vi "Read Image Blocks (SubVI).vi"(8 "Num of Image Blocks":i32, 10 "Image In":u8[][](array[numeric]), 11 "File REF In":refnum<file>) -> (2 "Image Out":u8[][](array[numeric]), 3 "File REF Out":refnum<file>)   [LabVIEW 2015]
panel:
  out "Image":T1(plugin-control)
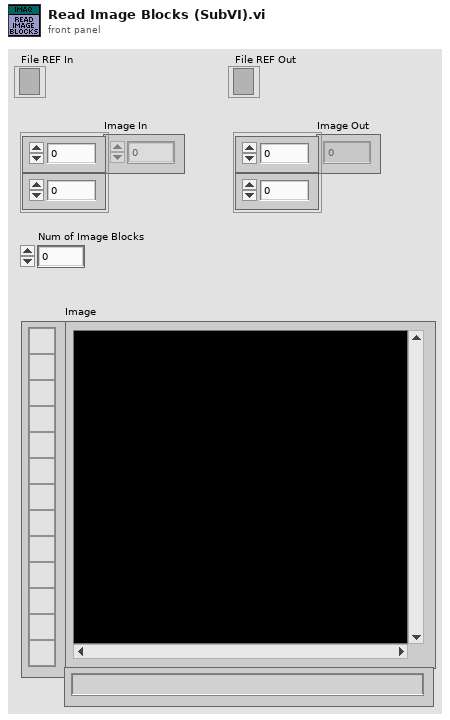
[diagram p1: front panel]
types:
  T1 = typedef "IMAQ Image.ctl" = refnum<image>
  T2 = enum16{"big-endian, network order", "native, host order", "little-endian"}
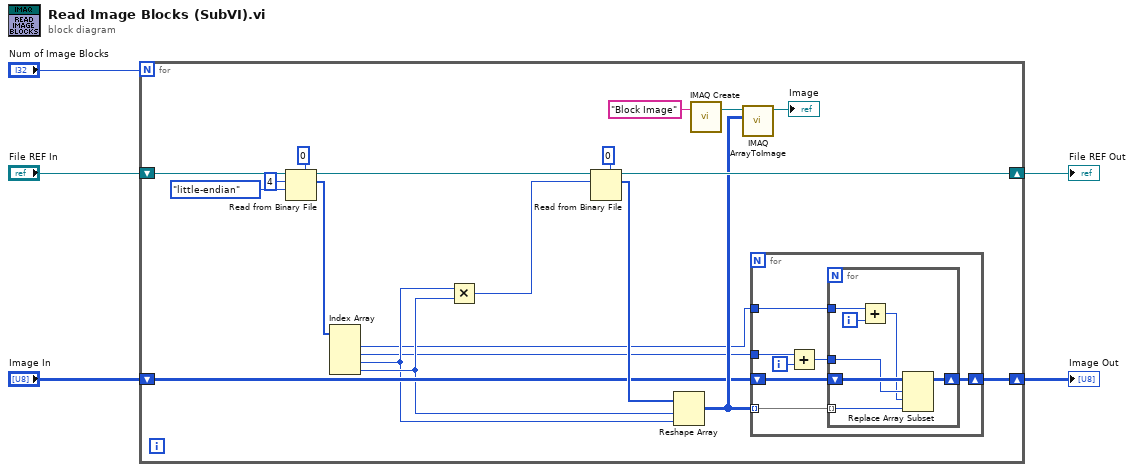
[diagram p0: block diagram]
diagram:
  n1 = for {
    N: "Num of Image Blocks" -> [_]
    shift-right: [w15] -> w2
    shift-left: "File REF In" -> [w17]
    shift-right: [w16] -> w4
    shift-left: "Image In" -> [w10]
    n2 = Read from Binary File(5:0, 9:T2."little-endian" ("byte order (0:big-endian, network order)"), 10:4 ("count (1)"), 11:w17) -> (2:w19:i32[], 3:w23:refnum<file>)  [unwired: 2 in, 2 out]
    n3 = Index Array(array=w19) -> (element #1=w6:i32, element #2=w7:i32, element #3=w8:i32, element #4=w9:i32)  [unwired: 4 in]
    n4 = Multiply(x=w8, y=w9) -> (x*y=w24:i32)
    n5 = Read from Binary File(5:u8 0, 10:w24, 11:w23) -> (2:w25:u8[], 3:w15:refnum<file>)  [unwired: 3 in, 2 out]
    n6 = Reshape Array(w25, w9, w8) -> (w11:u8[][])
    n7 = call "IMAQ Create"("Image Name"="Block Image") -> ("New Image"=w13:T1)  [unwired: 4 in, 1 out]
    n8 = call "IMAQ ArrayToImage"("Image Pixels (U8)"=w11, "Image"=w13) -> ("Image Out"=→"Image":T1)  [unwired: 8 in, 1 out]
    n9 = for {
      shift-right: [w31] -> w16
      shift-left: w10 -> [w32]
      tunnel: w7 -> [w30]
      tunnel: w11 -> [w27] mode=indexing
      tunnel: w6 -> [w26]
      i -> [w28]
      n10 = Add(x=w30, y=w28) -> (x+y=w29:i32)
      n11 = for {
        tunnel: w29 -> [w34]
        tunnel: w27 -> [w37] mode=indexing
        shift-right: [w38] -> w31
        shift-left: w32 -> [w39]
        tunnel: w26 -> [w35]
        i -> [w36]
        n12 = Add(x=w35, y=w36) -> (x+y=w33:i32)
        n13 = Replace Array Subset(array=w39, new element=w37, index (row)=w34, index (col)=w33) -> (w38:u8[][])
      }
    }
  }
  "Image Out" <- w4
  "File REF Out" <- w2
